vi "slscsl_initialize.vi"(7 "deviceIdentifier":string, 8 "error in (no error)":errorcluster, 9 "top file path":path, 10 "shw file path":path, 11 "topology Name":string) -> (0 "error out":errorcluster, 3 "slscsl out":refnum<class "slscsl.lvclass">)   [LabVIEW 2016, in "SLSC Switch.lvlib" / "slscsl.lvclass"]
uses:
  slscsl.lvclass
  slscsl.lvclass/slscsl.ctl
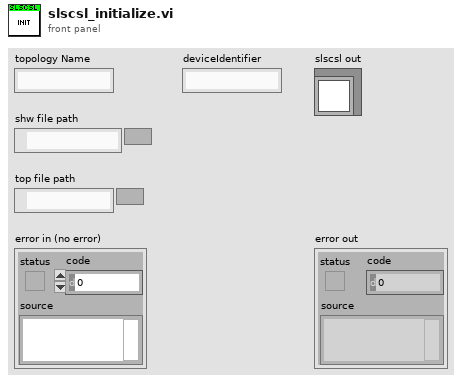
[diagram p1: front panel]
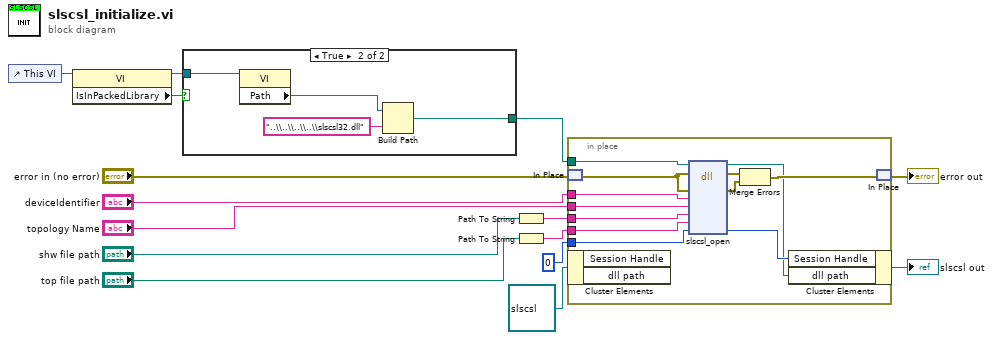
[diagram p0: block diagram]
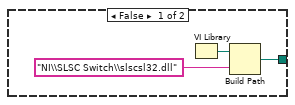
[diagram p2: hidden frame]
diagram:
  n1 = control-ref of="This VI"() -> (w7:refnum<vi>)
  n2 = property class="VI"(reference=w7) -> (reference out=w5:refnum<vi>, "IsInPackedLibrary"=w6:bool)  [unwired: 1 in, 1 out]
  n3 = case shown="True" w6 {
    tunnel: w5 -> [_ w20]
    tunnel: [w16 w21] -> w4
    frame False {
      n4 = VI Library() -> (path=w18:path)
      n5 = Build Path(base path=w18, name or relative path="NI\\SLSC Switch\\slscsl32.dll") -> (appended path=w16:path)
    }
    frame True {
      n6 = property class="VI"(reference=w20) -> ("Path"=w19:path)  [unwired: 1 in, 2 out]
      n7 = Build Path(base path=w19, name or relative path="..\\..\\..\\..\\slscsl32.dll") -> (appended path=w21:path)
    }
  }
  n8 = Path To String(path="shw file path") -> (string=w11:string)
  n9 = Path To String(path="top file path") -> (string=w12:string)
  n10 = in-place {
    in-place-border: "deviceIdentifier" -> [w34]
    in-place-border: u64 0 ("sessionHandlePtr") -> [w33]
    in-place-border: w12 -> [w32]
    in-place-border: w11 -> [w31]
    in-place-border: "topology Name" -> [w25]
    in-place-border: w4 -> [w24]
    n11 = in-place-match #1("error in (no error)") -> (w27:errorcluster)
    n12 = in-place-cluster #2(refnum<class "slscsl.lvclass"> refnum ("Route Manager out")) -> ()  [unwired: 2 out]
    n13 = dll-call lib="slscsl*.dll" fn="slscsl_open"(path in=w24, error in=w27, "errorCluster"=w27, "deviceIdentifier"=w34, "topologyName"=w25, "shwFilePath"=w31, "topFilePath"=w32, "sessionHandlePtr"=w33) -> (path out=w23:path, error out=w29:errorcluster, "errorCluster"=w28:errorcluster, "sessionHandlePtr"=w30:u64)  [unwired: 6 in]
    n14 = Merge Errors(w29, w28) -> (w26:errorcluster)
    n15 = in-place-cluster #2("Session Handle"=w30, "dll path"=w23) -> (→"slscsl out":refnum<class "slscsl.lvclass">)
    n16 = in-place-match #1(w26) -> (→"error out":errorcluster)
  }
